vi "Module Init.vi"(8 "error in (no error)":errorcluster, 11 "PluginGUI in":refnum<class "PluginGUI.lvclass">) -> (0 "error out":errorcluster, 3 "PluginGUI out":refnum<class "PluginGUI.lvclass">)   [LabVIEW 2020, in "VolatusGUI.lvlib" / "PluginGUI.lvclass"]
uses:
  PluginGUI.lvclass
  C:/dev/lv20CE/relink/lv-volatus/Volatus/Module/Module.lvclass
  Volatus/Module/Module.lvclass/Module.ctl
  Volatus/MessageQ/MessageQ.lvclass/MessageQ.ctl
  Volatus/Module/Self Q.vi
  Volatus/MessageQ/Send.vi
  PluginGUI.lvclass/PluginGUI.ctl
  Volatus/Module/Module.lvclass
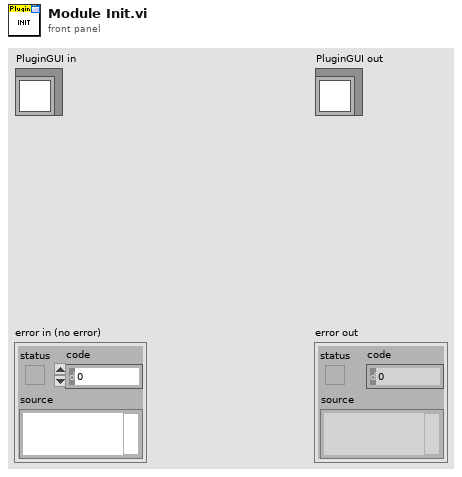
[diagram p1: front panel]
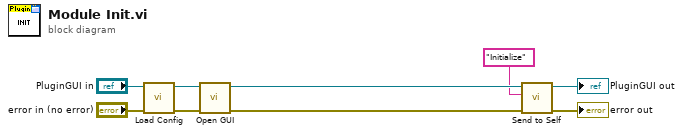
[diagram p0: block diagram]
diagram:
  n1 = call "Load Config.vi"("error in (no error)"="error in (no error)", "PluginGUI in"="PluginGUI in") -> ("error out"=w8:errorcluster, "PluginGUI out"=w6:refnum<class "PluginGUI.lvclass">)  [unwired: 8 in]
  n2 = call "Open GUI.vi"("error in (no error)"=w8, "PluginGUI in"=w6) -> ("error out"=w4:errorcluster, "PluginGUI out"=w5:refnum<class "PluginGUI.lvclass">)  [unwired: 8 in]
  n3 = call "Send to Self.vi"("error in (no error)"=w4, "Message ID"="Initialize", "Module in"=w5) -> ("error out"=→"error out":errorcluster, "Module out"=→"PluginGUI out":refnum<class "PluginGUI.lvclass">)  [unwired: 7 in]
